vi "randomTest.vi"() -> ()   [LabVIEW 2015]
panel:
  out "concatenated string":string
  out "Array 2":i32[](array[numeric])
  out "Array":string[](array[string])
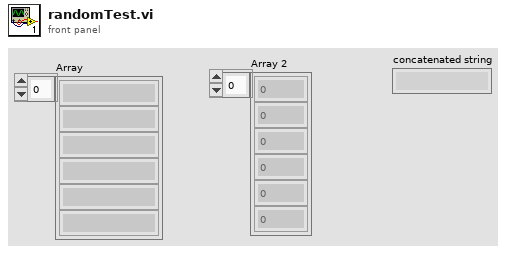
[diagram p1: front panel]
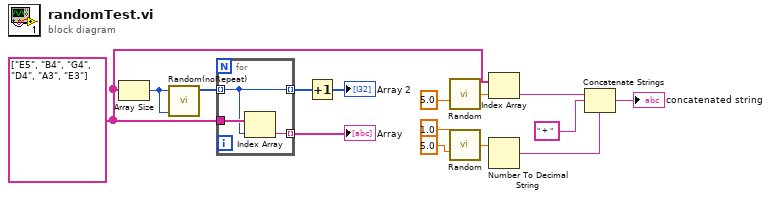
[diagram p0: block diagram]
diagram:
  w9 = string[] ["E5", "B4", "G4", "D4", "A3", "E3"]
  n1 = Array Size(array=w9) -> (size(s)=w1:i32)
  n2 = call <userlib>:"Random(noRepeat).vi"("Max"=w1, "輸入點數"=w1) -> ("Array"=w14:i32[])  [unwired: 9 in]
  n3 = for {
    tunnel: w14 -> [w16] mode=indexing
    tunnel: [w18] -> w15 mode=indexing
    tunnel: w9 -> [w17]
    tunnel: [w16] -> w13 mode=indexing
    n4 = Index Array(array=w17, index=w16) -> (element=w18:string)
  }
  "Array" <- w15
  n5 = Increment(x=w13) -> (x+1=→"Array 2":i32[])
  n6 = call <userlib>:"Random.vi"("Max"=5.0) -> ("Random"=w10:dbl)  [unwired: 14 in]
  n7 = call <userlib>:"Random.vi"("Min(0)"=1.0, "Max"=5.0) -> ("Random"=w8:dbl)  [unwired: 13 in]
  n8 = Index Array(array=w9, index=w10) -> (element=w7:string)
  n9 = Number To Decimal String(number=w8) -> (decimal integer string=w3:string)  [unwired: 1 in]
  n10 = Concatenate Strings(w7, " + ", w3) -> (→"concatenated string":string)
